vi "GetBounds.vi"(0 "XRef":T6, 1 "State In":T4) -> (14 "Bounds":T2, 15 "Fatal Error Out":T1)   [LabVIEW 2015, in "LVJSON.lvlib" / "Set Object Parameters.xnode"]
uses:
  Set Object Parameters.xnode
  <vilib>/XNodeSupport/XNodeXNodeRef.ctl
  State.ctl
  Get Object Parameters/Parameter.ctl
  <vilib>/XNodeSupport/XNodeBounds.ctl
  <vilib>/XNodeSupport/XNodeInt.ctl
  <vilib>/XNodeSupport/XNodeErrorCluster.ctl
  offsets.vi
  <vilib>/XNodeSupport/NI_XNodeSupport.lvlib
  Shared/Shared.lvlib
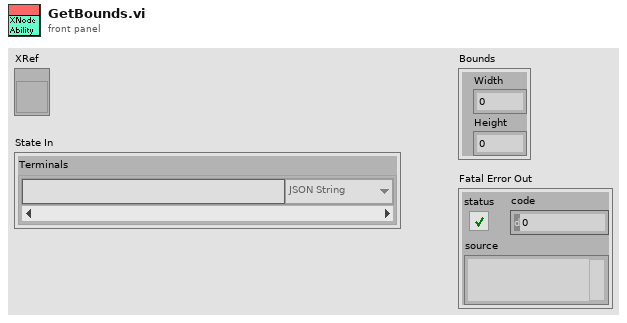
[diagram p1: front panel]
types:
  T1 = typedef "NI_XNodeSupport.lvlib/XNodeErrorCluster.ctl" = errorcluster
  T2 = typedef "NI_XNodeSupport.lvlib/XNodeBounds.ctl" = cluster{"Width":T3, "Height":T3}
  T3 = typedef "NI_XNodeSupport.lvlib/XNodeInt.ctl" = i32
  T4 = typedef "LVJSON.lvlib/Set Object Parameters.xnode/State.ctl" = cluster{"Terminals":T5[]}
  T5 = typedef "LVJSON.lvlib/Shared.lvlib/Parameter.ctl" = cluster{"Parameter Name":string, "JSON Type":enum16{"JSON String", "JSON Numeric", "JSON Boolean", "JSON", "JSON Object", "JSON Array", "String Value", "Numeric Value", "Boolean Value"}}
  T6 = typedef "NI_XNodeSupport.lvlib/XNodeXNodeRef.ctl" = refnum<vi>
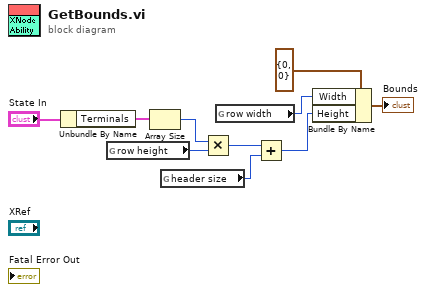
[diagram p0: block diagram]
diagram:
  n1 = Unbundle By Name("State In") -> ("Terminals"=w9:T5[])
  n2 = global read "offsets.vi" "row height"() -> (w2:i16)
  n3 = Array Size(array=w9) -> (size(s)=w7:i32)
  n4 = global read "offsets.vi" "header size"() -> (w3:i16)
  n5 = Multiply(x=w7, y=w2) -> (x*y=w5:i32)
  n6 = global read "offsets.vi" "row width"() -> (w1:i16)
  n7 = Add(x=w5, y=w3) -> (x+y=w4:i32)
  n8 = Bundle By Name(cluster=T2 {"Width"=0, "Height"=0} ("Bounds"), "Width"=w1, "Height"=w4) -> (→"Bounds":T2)
